vi "Configure AIN U3.vi"(4 "Binary":bool, 6 "longSettling":bool, 8 "error in":errorcluster, 10 "quickSample":bool, 11 "Handle In":i32) -> (0 "error out":errorcluster, 3 "Handle Out":i32)   [LabVIEW 2021]
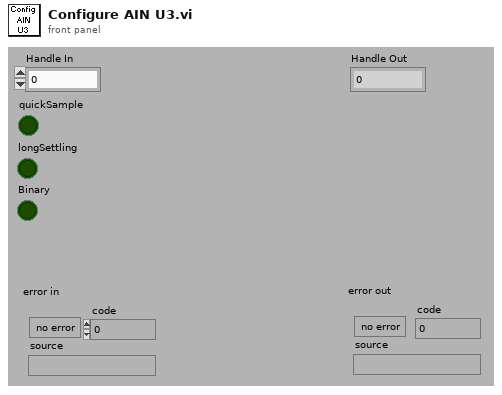
[diagram p1: front panel]
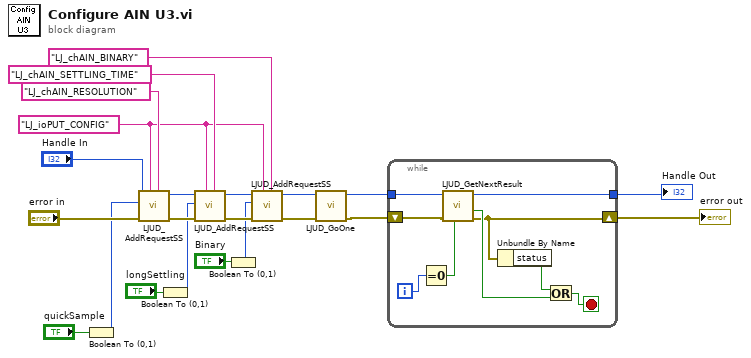
[diagram p0: block diagram]
diagram:
  w13 = "LJ_ioPUT_CONFIG" ("IOType")
  n1 = Boolean To (0,1)(Boolean="quickSample") -> (0, 1=w10:i16)
  n2 = call "LJUD_AddRequestSS.vi"("Channel"="LJ_chAIN_RESOLUTION" ("IOType"), "IOType"=w13, "error in"="error in", "Value"=w10, "Handle In"="Handle In") -> ("error out"=w18:errorcluster, "Handle Out"=w20:i32)  [unwired: 5 in]
  n3 = Boolean To (0,1)(Boolean="longSettling") -> (0, 1=w4:i16)
  n4 = call "LJUD_AddRequestSS.vi"("Channel"="LJ_chAIN_SETTLING_TIME" ("IOType"), "IOType"=w13, "error in"=w18, "Value"=w4, "Handle In"=w20) -> ("error out"=w17:errorcluster, "Handle Out"=w19:i32)  [unwired: 5 in]
  n5 = Boolean To (0,1)(Boolean="Binary") -> (0, 1=w8:i16)
  n6 = call "LJUD_AddRequestSS.vi"("Channel"="LJ_chAIN_BINARY" ("IOType"), "IOType"=w13, "error in"=w17, "Value"=w8, "Handle In"=w19) -> ("error out"=w1:errorcluster, "Handle Out"=w2:i32)  [unwired: 5 in]
  n7 = call "LJUD_GoOne.vi"("error in"=w1, "Handle In"=w2) -> ("error out"=w7:errorcluster, "Handle Out"=w21:i32)  [unwired: 8 in]
  n8 = while {
    shift-left: w7 -> [w24]
    shift-right: [w23] -> w6
    tunnel: [w27] -> w22
    tunnel: w21 -> [w29]
    i -> [w26]
    stop <- w31 stop-if-true
    n9 = Equal To 0?(x=w26) -> (x = 0?=w30:bool)
    n10 = call "LJUD_GetNextResult.vi"("GetFirst"=w30, "error in"=w24, "Handle In"=w29) -> ("error out"=w23:errorcluster, "LJE_NO_MORE_DATA_AVAILABLE"=w25:bool, "Handle Out"=w27:i32)  [unwired: 3 in, 3 out]
    n11 = Unbundle By Name(w23) -> ("status"=w28:bool)
    n12 = Or(x=w28, y=w25) -> (x .or. y?=w31:bool)
  }
  "Handle Out" <- w22
  "error out" <- w6
